vi "Back_Ket_Zero.vi"(8 "error in":errorcluster, 10 "VD_Supply":dbl=16.0, 11 "VISA Ket":refnum<visa-resource-name>) -> (0 "error out":errorcluster, 3 "VISA Ket":refnum<visa-resource-name>)   [LabVIEW 2012]
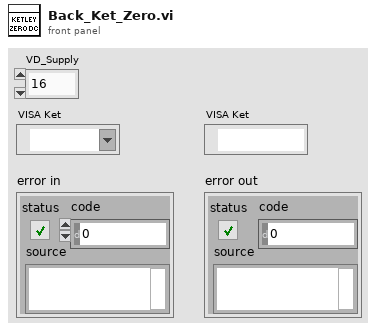
[diagram p1: front panel]
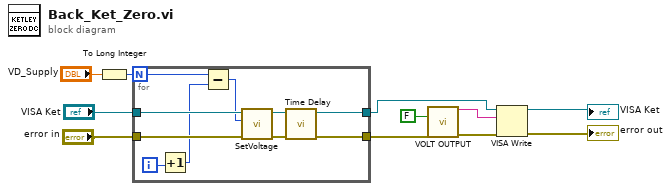
[diagram p0: block diagram]
diagram:
  n1 = To Long Integer(number="VD_Supply") -> (32bit integer=w8:i32)
  n2 = for {
    N: w8 -> [w15]
    tunnel: "VISA Ket" -> [w20]
    tunnel: "error in" -> [w19]
    tunnel: [w18] -> w3
    tunnel: [w16] -> w4
    i -> [w14]
    n3 = Increment(x=w14) -> (x+1=w12:i32)
    n4 = Subtract(x=w15, y=w12) -> (x-y=w13:i32)
    n5 = call "SetVoltage.vi"("error in"=w19, "Input Voltage"=w13, "VISA Ket"=w20) -> ("error out"=w17:errorcluster, "VISA Ket"=w18:refnum<visa-resource-name>)  [unwired: 7 in]
    n6 = call "Time Delay"("error in (no error)"=w17) -> ("error out"=w16:errorcluster)  [unwired: 10 in]
  }
  n7 = call "VOLT OUTPUT"("VOLTOUTPUT"=FALSE ("On?"), "error in (no error)"=w4) -> ("Result"=w5:string, "error out"=w6:errorcluster)  [unwired: 12 in]
  n8 = VISA Write(VISA resource name=w3, write buffer=w5, error in (no error)=w6) -> (VISA resource name out=→"VISA Ket":refnum<visa-resource-name>, error out=→"error out":errorcluster)  [unwired: 1 out]
